vi "Selecting the highest pixel.vi"(8 "error in":errorcluster, 10 "Column Number":i32, 11 "Value of End Pixel":i32) -> (0 "error out":errorcluster)   [LabVIEW 2016]
uses:
  <vilib>/userdefined/High Color/IMAQdx.ctl
  <vilib>/vision/driver/NI_Vision_Acquisition_Software.lvlib
panel:
  out "Pixel Value":dbl
  out "Maximum Gradient 3":u8
  out "Maximum Gradient 2":u8
  out "Maximum Gradient":u8
  out "Pixel Value 3":i32
  out "Pixel Value 2":i32
  out "Pixel Value":i32
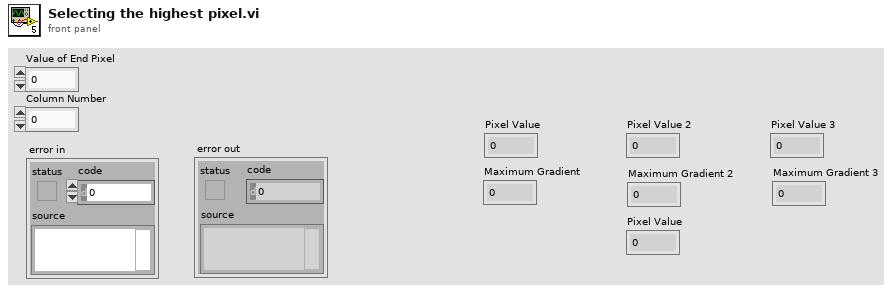
[diagram p1: front panel]
types:
  T1 = typedef "IMAQdx.ctl" = refnum<k21>
  T2 = typedef "IMAQ Image.ctl" = refnum<image>
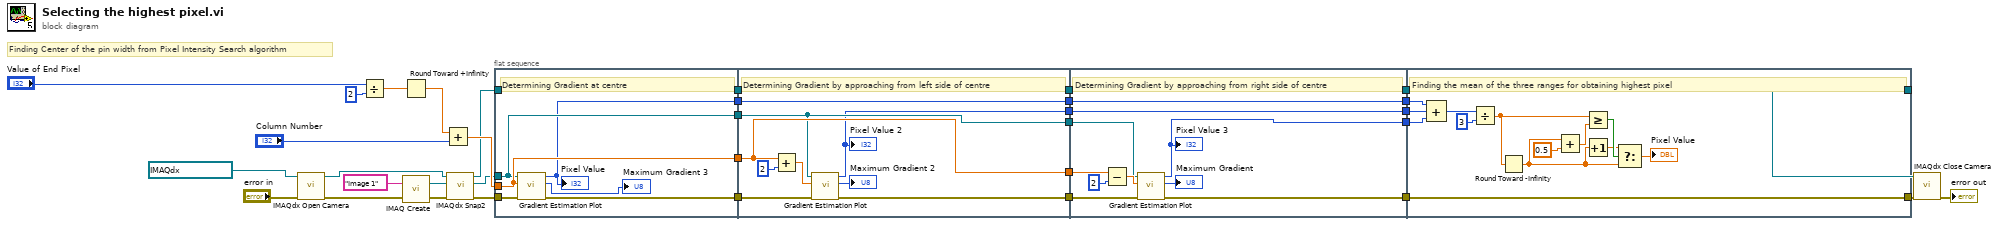
[diagram p0: block diagram]
diagram:
  # "Finding Center of the pin width from Pixel Intensity Search algorithm"
  n1 = call <vilib>:"IMAQdx Open Camera.vi"("error in"="error in", "Session In"=T1 "acA780-75gc") -> ("error out"=w26:errorcluster, "Session Out"=w21:T1)  [unwired: 8 in]
  n2 = Divide(x="Value of End Pixel", y=2) -> (x/y=w33:dbl)
  n3 = Round Toward +Infinity(x=w33) -> (ceil(x): smallest int >= x=w31:dbl)
  n4 = call "IMAQ Create"("Image Name"="Image 1", "error in (no error)"=w26) -> ("New Image"=w25:T2, "error out"=w27:errorcluster)  [unwired: 3 in]
  n5 = Add(x=w31, y="Column Number") -> (x+y=w30:dbl)
  n6 = call <vilib>:"IMAQdx Snap2.vi"("error in"=w27, "Image In"=w25, "Session In"=w21) -> ("error out"=w16:errorcluster, "Image Out"=w11:T2, "Session Out"=w20:T1)  [unwired: 6 in]
  n7 = flat-sequence {
    tunnel: w30 -> [w42]
    tunnel: [w42] -> w29
    tunnel: w20 -> [w41]
    tunnel: [w41] -> w18
    tunnel: w16 -> [w40]
    tunnel: [w39] -> w15
    tunnel: w11 -> [w38]
    tunnel: [w38] -> w10
    tunnel: [w36] -> w4
    tunnel: w29 -> [w51]
    tunnel: [w51] -> w28
    tunnel: [w49] -> w19
    tunnel: w18 -> [w49]
    tunnel: w15 -> [w48]
    tunnel: [w47] -> w14
    tunnel: w10 -> [w46]
    tunnel: [w46] -> w9
    tunnel: [w44] -> w5
    tunnel: w4 -> [w44]
    tunnel: [w43] -> w2
    tunnel: w28 -> [w63]
    tunnel: w19 -> [w60]
    tunnel: w14 -> [w59]
    tunnel: w9 -> [w57]
    tunnel: [w60] -> w8
    tunnel: [w58] -> w7
    tunnel: [w55] -> w6
    tunnel: w5 -> [w55]
    tunnel: [w54] -> w3
    tunnel: w2 -> [w54]
    tunnel: [w53] -> w1
    tunnel: [w76] -> w13
    tunnel: [w77] -> w17
    tunnel: w8 -> [w77]
    tunnel: w7 -> [w76]
    tunnel: w6 -> [w75]
    tunnel: w3 -> [w74]
    tunnel: w1 -> [w73]
    frame #0 {
      # "Determining Gradient at centre"
      n8 = call "Gradient Estimation Plot.vi"("error in (no error)"=w40, "Pixel Column Number"=w42, "Image"=w38) -> ("error out"=w39:errorcluster, "Maximum Gradient"=→"Maximum Gradient 3":u8, "Pixel Value"=w36:i32)  [unwired: 4 in, 2 out]
      "Pixel Value" <- w36
    }
    frame #1 {
      # "Determining Gradient by approaching from left side of centre"
      n9 = Add(x=w51, y=2) -> (x+y=w52:dbl)
      n10 = call "Gradient Estimation Plot.vi"("error in (no error)"=w48, "Pixel Column Number"=w52, "Image"=w46) -> ("error out"=w47:errorcluster, "Maximum Gradient"=→"Maximum Gradient 2":u8, "Pixel Value"=w43:i32)  [unwired: 4 in, 2 out]
      "Pixel Value 2" <- w43
    }
    frame #2 {
      # "Determining Gradient by approaching from right side of centre"
      n11 = Subtract(x=w63, y=2) -> (x-y=w61:dbl)
      n12 = call "Gradient Estimation Plot.vi"("error in (no error)"=w59, "Pixel Column Number"=w61, "Image"=w57) -> ("error out"=w58:errorcluster, "Maximum Gradient"=→"Maximum Gradient":u8, "Pixel Value"=w53:i32)  [unwired: 4 in, 2 out]
      "Pixel Value 3" <- w53
    }
    frame #3 {
      # "Finding the mean of the three ranges for obtaining highest pixel"
      n13 = Compound Arithmetic op=ADD(w75, w74, w73) -> (w72:i32)
      n14 = Divide(x=w72, y=3) -> (x/y=w70:dbl)
      n15 = Round Toward -Infinity(1:w70) -> (0:w66:dbl)
      n16 = Add(x=w66, y=0.5) -> (x+y=w65:dbl)
      n17 = Greater Or Equal?(x=w70, y=w65) -> (x >= y?=w69:bool)
      n18 = Increment(x=w66) -> (x+1=w68:dbl)
      n19 = Select(t=w68, s=w69, f=w66) -> (s? t:f=→"Pixel Value":dbl)
    }
  }
  n20 = call <vilib>:"IMAQdx Close Camera.vi"("error in"=w13, "Session In"=w17) -> ("error out"=→"error out":errorcluster)  [unwired: 9 in]
